vi "gateway记录.vi"() -> ()   [LabVIEW 2012]
panel:
  out "保存的路径":path=path "E:/大学文档/大四下/毕设/wsn_project2/13_050400.tdms"
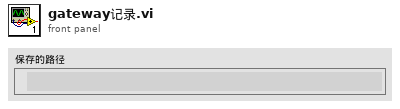
[diagram p1: front panel]
types:
  T1 = cluster{i32, enum16{"温度", "亮度", "电量", "连接质量"}, sgl}
  T2 = enum16{"open", "open or create", "create or replace", "create", "open (read-only)"}
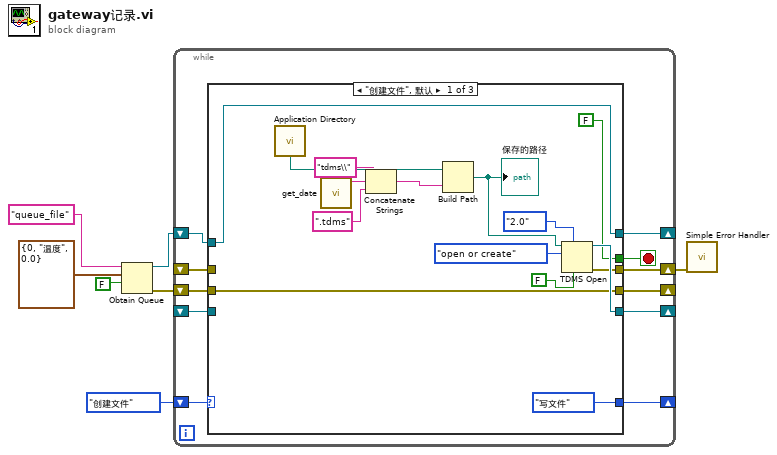
[diagram p0: block diagram]
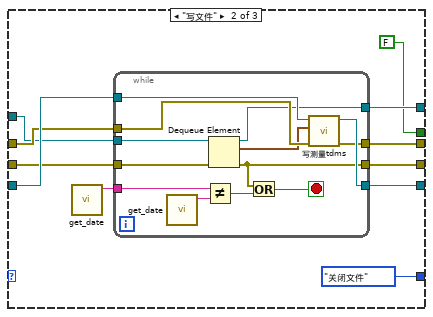
[diagram p2: hidden frame]
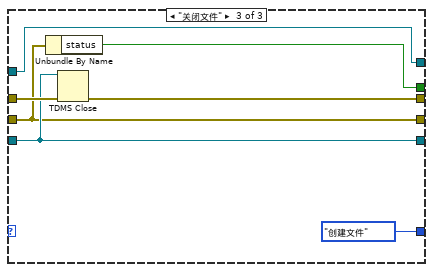
[diagram p3: hidden frame]
diagram:
  n1 = Obtain Queue(name (unnamed)="queue_file" ("名称（未命名）"), element data type=T1 {0, enum."温度", 0.0}, create if not found? (T)=FALSE ("如未找到是否创建？(T)")) -> (queue out=w3:refnum<queue>, error out=w4:errorcluster)  [unwired: 2 in, 1 out]
  n2 = while {
    shift-right: [w18] -> _
    shift-left: _ -> [w16]
    shift-right: [w17] -> w1
    shift-left: _ -> [w15]
    shift-right: [w13] -> _
    shift-left: enum16{"创建文件", "写文件", "关闭文件"}."创建文件" -> [w14]
    shift-right: [w11] -> _
    shift-left: w4 -> [w12]
    shift-right: [w9] -> _
    shift-left: w3 -> [w10]
    stop <- w8 stop-if-true
    n3 = case shown="\"创建文件\", 默认" w14 {
      tunnel: [w30 w40 w63] -> w18
      tunnel: [w29 w39 w62] -> w17
      tunnel: [enum16{"创建文件", "写文件", "关闭文件"}."写文件" enum16{"创建文件", "写文件", "关闭文件"}."关闭文件" enum16{"创建文件", "写文件", "关闭文件"}."创建文件"] -> w13
      tunnel: w16 -> [_ w44 w63]
      tunnel: w15 -> [_ w43 w64]
      tunnel: w12 -> [w21 w38 w59]
      tunnel: [w21 w37 w59] -> w11
      tunnel: w10 -> [w22 w36 w60]
      tunnel: [w22 w35 w60] -> w9
      tunnel: [FALSE ("status") FALSE ("status") w58] -> w8
      frame "创建文件", Default {
        n4 = call <vilib>:"Application Directory.vi"() -> ("Application Directory"=w28:path)
        n5 = call "get_date.vi"() -> ("日期/时间字符串"=w27:string)  [unwired: 11 in]
        n6 = Concatenate Strings("tdms\\" ("字符串"), w27, ".tdms" ("字符串")) -> (w25:string)
        n7 = Build Path(base path=w28, name or relative path=w25) -> (appended path=w24:path)
        "保存的路径" <- w24
        n8 = TDMS Open(6:FALSE ("禁用缓冲？(T)"), 7:enum16{"1.0", "2.0"}."2.0" ("文件格式版本(2.0)"), 10:T2."open or create" ("操作(0:open)"), 11:w24) -> (0:w29:errorcluster, 3:w30:refnum<k34>)  [unwired: 2 in]
      }
      frame "写文件" {
        n9 = call "get_date.vi"() -> ("日期/时间字符串"=w42:string)  [unwired: 11 in]
        n10 = while {
          tunnel: w44 -> [w55]
          tunnel: w43 -> [w54]
          tunnel: w42 -> [w57]
          tunnel: [w53] -> w40
          tunnel: [w52] -> w39
          tunnel: w38 -> [w50]
          tunnel: [w47] -> w37
          tunnel: w36 -> [w49]
          tunnel: [w48] -> w35
          stop <- w45 stop-if-true
          n11 = call "get_date.vi"() -> ("日期/时间字符串"=w56:string)  [unwired: 11 in]
          n12 = Not Equal?(x=w57, y=w56) -> (x != y?=w46:bool)
          n13 = Dequeue Element(queue=w49, error in (no error)=w50) -> (queue out=w48:refnum<queue>, element=w51:T1, error out=w47:errorcluster)  [unwired: 1 in, 1 out]
          n14 = Or(x=w47, y=w46) -> (x .or. y?=w45:bool)
          n15 = call "写测量tdms.vi"("错误输入（无错误）"=w54, "消息"=w51, "引用句柄输入"=w55) -> ("错误输出"=w52:errorcluster, "tdms文件输出"=w53:refnum<k34>)  [unwired: 7 in]
        }
      }
      frame "关闭文件" {
        n16 = Unbundle By Name(w59) -> ("status"=w58:bool)
        n17 = TDMS Close(8:w64, 11:w63) -> (0:w62:errorcluster)  [unwired: 1 out]
      }
    }
  }
  n18 = call <vilib>:"Simple Error Handler.vi"("error in (no error)"=w1) -> ()  [unwired: 4 in, 5 out]
